vi "IsEquivalentEXT.vi"(3 "Digits":i32=6 caption="Digits (6)", 4 "Y":ext, 5 "X":ext) -> (1 "Equivalent?":bool)   [LabVIEW 2017, in "GPComparison.lvlib"]
doc: "<B>X</B> and <B>Y</B> are deemed <B>Equivalent?</B> if they are equal to within the specified number of decimal <B>Digits</B>.\n\nEqual in this case is defined as within Machine Epsilon of each other after rounding to number of <B>Digits</B>. Machine Epsilon is the smallest value respresentable for the given data type on this particular computer.\n\nTwo NaNs (Not-A-Number) are deemed equivalent, although they are not equal per the IEEE 754 standard.\n\n<B>Note</B> This VI uses the default IEEE 754 round-half-to-even rounding mode. A negative number of <B>Digits</B> means rounding to ones, tens, hundreds, etc.\n\nThis VI is inlined.\n\nSteen Schmidt\nGPower\n22/10 2016"
uses:
  GPComparison.lvlib
panel:
  # "Copyright © 2016\nGPower\nSee enclosed license file for terms and conditions"
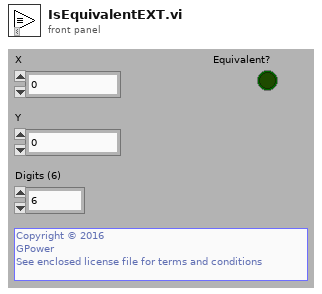
[diagram p1: front panel]
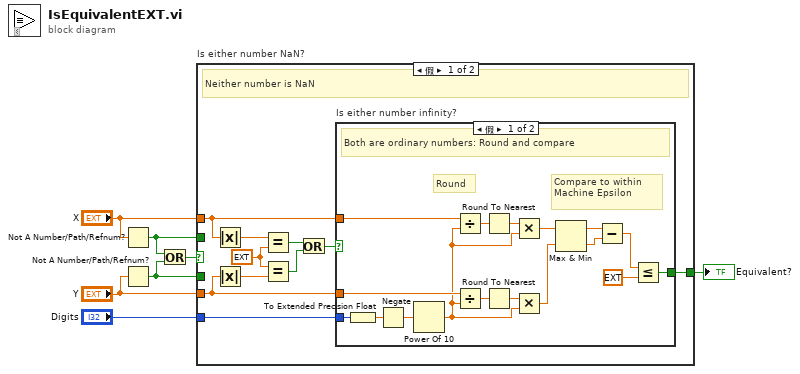
[diagram p0: block diagram]
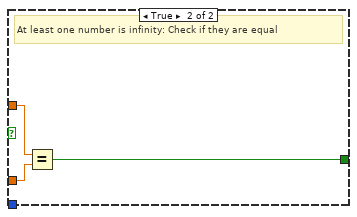
[diagram p2: hidden frame]
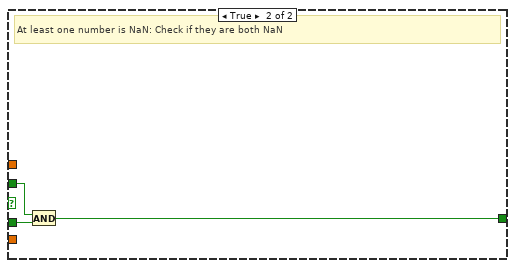
[diagram p3: hidden frame]
diagram:
  n1 = Not A Number/Path/Refnum?(number/path/refnum="X") -> (NaN/Path/Refnum?=w1:bool)
  n2 = Not A Number/Path/Refnum?(number/path/refnum="Y") -> (NaN/Path/Refnum?=w3:bool)
  n3 = Or(x=w1, y=w3) -> (x .or. y?=w2:bool)
  n4 = case "Is either number NaN?" shown="假" w2 {
    tunnel: "Digits" -> [w17 _]
    tunnel: "X" -> [w15 _]
    tunnel: "Y" -> [w13 _]
    tunnel: [w16 w39] -> w4
    tunnel: w3 -> [_ w38]
    tunnel: w1 -> [_ w40]
    frame False {
      w11 = ext inf
      # "Neither number is NaN"
      n5 = Absolute Value(x=w15) -> (abs(x)=w14:ext)
      n6 = Absolute Value(x=w13) -> (abs(x)=w12:ext)
      n7 = Equal?(x=w14, y=w11) -> (x = y?=w10:bool)
      n8 = Equal?(x=w11, y=w12) -> (x = y?=w9:bool)
      n9 = Or(x=w10, y=w9) -> (x .or. y?=w8:bool)
      n10 = case "Is either number infinity?" shown="假" w8 {
        tunnel: w17 -> [w34 _]
        tunnel: w15 -> [w33 w37]
        tunnel: w13 -> [w32 w35]
        tunnel: [w25 w36] -> w16
        frame False {
          # "Compare to within\nMachine Epsilon"
          # "Round"
          # "Both are ordinary numbers: Round and compare"
          n11 = To Extended Precision Float(1:w34) -> (0:w21:ext)
          n12 = Negate(x=w21) -> (-x=w22:ext)
          n13 = Power Of 10(x=w22) -> (10^x=w18:ext)
          n14 = Divide(x=w33, y=w18) -> (x/y=w19:ext)
          n15 = Divide(x=w32, y=w18) -> (x/y=w24:ext)
          n16 = Round To Nearest(number=w19) -> (nearest integer value=w20:ext)
          n17 = Round To Nearest(number=w24) -> (nearest integer value=w23:ext)
          n18 = Multiply(x=w20, y=w18) -> (x*y=w27:ext)
          n19 = Multiply(x=w23, y=w18) -> (x*y=w26:ext)
          n20 = Max & Min(x=w27, y=w26) -> (max(x,y)=w31:ext, min(x,y)=w30:ext)
          n21 = Subtract(x=w31, y=w30) -> (x-y=w29:ext)
          n22 = Less Or Equal?(x=w29, y=ext 1.0842021724855044e-19) -> (x <= y?=w25:bool)
        }
        frame True {
          # "At least one number is infinity: Check if they are equal"
          n23 = Equal?(x=w37, y=w35) -> (x = y?=w36:bool)
        }
      }
    }
    frame True {
      # "At least one number is NaN: Check if they are both NaN"
      n24 = And(x=w40, y=w38) -> (x .and. y?=w39:bool)
    }
  }
  "Equivalent?" <- w4
